vi "Class Variant 2 Cluster Variant.vi"(8 "error in (no error)":errorcluster, 10 "User VI Ref":refnum<vi>, 11 "Variant":variant) -> (0 "error out":errorcluster, 3 "Control Value:Get":variant)   [LabVIEW 2023]
uses:
  <vilib>/Utility/Data Type/NI_Data Type.lvlib
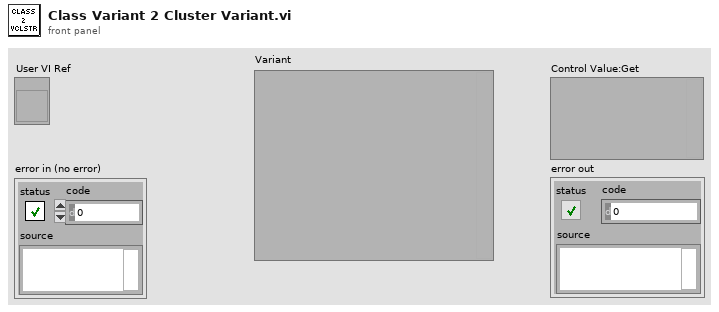
[diagram p1: front panel]
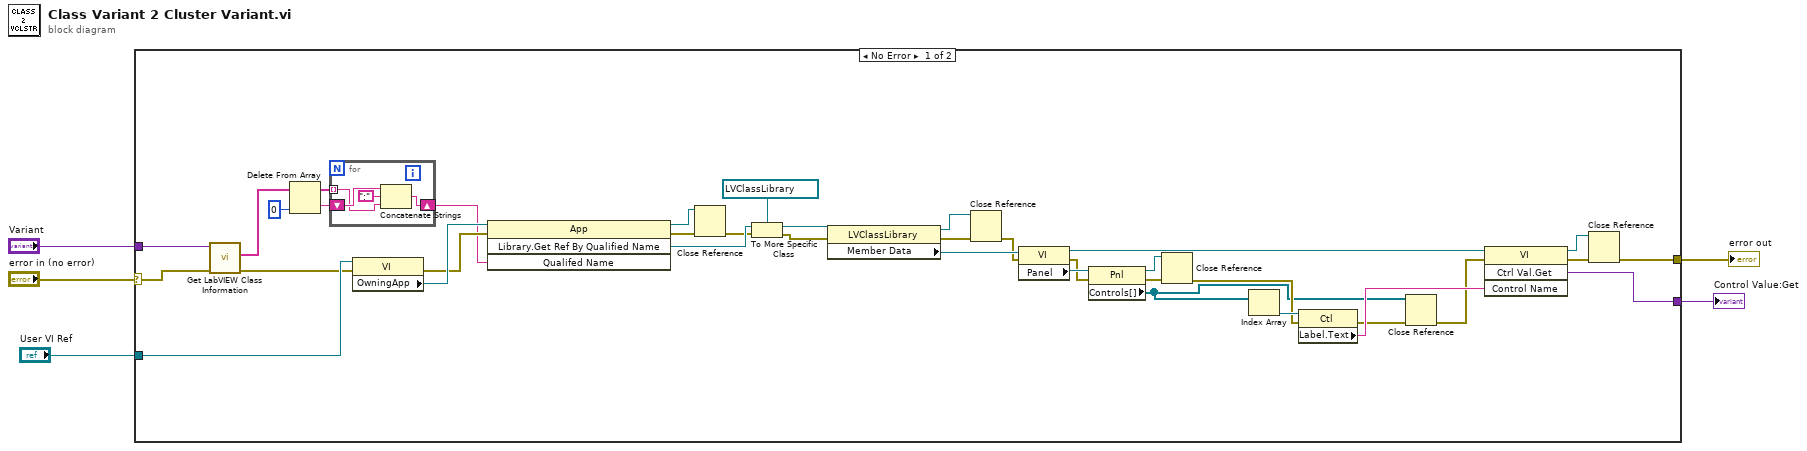
[diagram p0: block diagram]
diagram:
  n1 = case shown="No Error" "error in (no error)" {
    selector: "error in (no error)" -> [w38 w47]
    tunnel: "Variant" -> [w39 w48]
    tunnel: [w34 w48] -> w3
    tunnel: [w33 w47] -> w2
    tunnel: "User VI Ref" -> [w25 _]
    frame No Error {
      n2 = call <vilib>:"Get LabVIEW Class Information.vi"("error in (no error)"=w38, "variant"=w39) -> ("error out"=w23:errorcluster, "qualified LabVIEW class name"=w18:string[])  [unwired: 7 in, 1 out]
      n3 = Delete From Array(array=w18, index=0) -> (deleted portion=w15:string, array with subset deleted=w16:string[])  [unwired: 1 in]
      n4 = for {
        tunnel: w16 -> [w44] mode=indexing
        shift-right: [w45] -> w14
        shift-left: w15 -> [w46]
        n5 = Concatenate Strings(w46, ":" ("string"), w44) -> (w45:string)
      }
      n6 = property class="VI"(reference=w25, error in=w23) -> (error out=w22:errorcluster, "OwningApp"=w24:refnum<vi>)  [unwired: 1 out]
      n7 = invoke class="App" method="Library.Get Ref By Qualified Name"(reference=w24, error in=w22, "Qualifed Name"=w14) -> (reference out=w19:refnum<vi>, error out=w21:errorcluster, "Library.Get Ref By Qualified Name"=w28:refnum<vi>)  [unwired: 1 in, 1 out]
      n8 = Close Reference(reference=w19, error in (no error)=w21) -> (error out=w20:errorcluster)
      n9 = To More Specific Class(target class=refnum<vi> refnum ("reference"), reference=w28, error in=w20) -> (specific class reference=w26:refnum<vi>, error out=w27:errorcluster)
      n10 = property class="LVClassLibrary"(reference=w26, error in=w27) -> (reference out=w30:refnum<vi>, error out=w32:errorcluster, "Member Data"=w42:refnum<vi>)
      n11 = Close Reference(reference=w30, error in (no error)=w32) -> (error out=w31:errorcluster)
      n12 = property class="VI"(reference=w42, error in=w31) -> (reference out=w41:refnum<vi>, error out=w11:errorcluster, "Panel"=w13:refnum<vi>)
      n13 = property class="Pnl"(reference=w13, error in=w11) -> (reference out=w9:refnum<vi>, error out=w10:errorcluster, "Controls[]"=w6:refnum<vi>[])
      n14 = Close Reference(reference=w9, error in (no error)=w10) -> (error out=w8:errorcluster)
      n15 = Index Array(array=w6) -> (element=w12:refnum<vi>)  [unwired: 1 in]
      n16 = property class="Ctl"(reference=w12, error in=w8) -> (error out=w7:errorcluster, "Label.Text"=w40:string)  [unwired: 1 out]
      n17 = Close Reference(reference=w6, error in (no error)=w7) -> (error out=w37:errorcluster)
      n18 = invoke class="VI" method="Ctrl Val.Get"(reference=w41, error in=w37, "Control Name"=w40) -> (reference out=w35:refnum<vi>, error out=w36:errorcluster, "Get Control Value Variant"=w34:variant)  [unwired: 1 in, 1 out]
      n19 = Close Reference(reference=w35, error in (no error)=w36) -> (error out=w33:errorcluster)
    }
    frame Error {
    }
  }
  "Control Value:Get" <- w3
  "error out" <- w2
